vi "Get Excess TempProtection Setpoint.vi"(8 "error in (no error)":errorcluster, 11 "VISA resource name":refnum<visa-resource-name>) -> (0 "error out":errorcluster, 1 "ExcessTempProtection(out)":dbl, 3 "VISA resource name out":refnum<visa-resource-name>)   [LabVIEW 2018, in "JULABO DeviceDriver.lvlib"]
doc: "This VI returns the actual setting for the excess temperature protection. Please refer to operating manual for this safety setting."
uses:
  JULABO DeviceDriver.lvlib
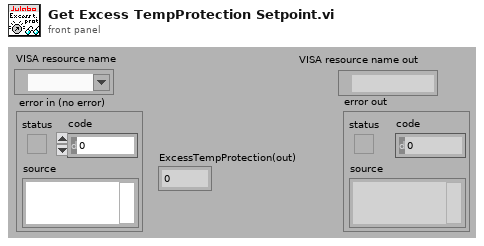
[diagram p1: front panel]
types:
  T1 = typedef "JULABO DeviceDriver.lvlib/InstrumentType.ctl" = enum8{"Default", "FC-Series", "HT30/HT60", "LC4"}
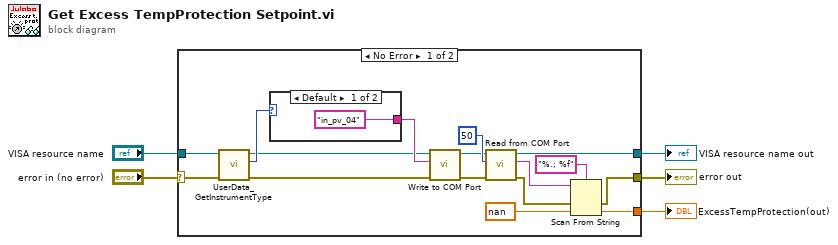
[diagram p0: block diagram]
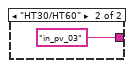
[diagram p2: hidden frame]
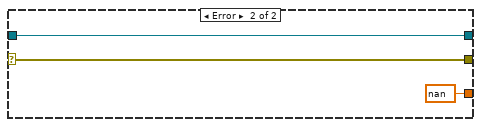
[diagram p3: hidden frame]
diagram:
  n1 = case shown="No Error" "error in (no error)" {
    selector: "error in (no error)" -> [w6 w25]
    tunnel: "VISA resource name" -> [w7 w26]
    tunnel: [w18 w25] -> w4
    tunnel: [w17 w26] -> w3
    tunnel: [w15 nan] -> w1
    frame No Error {
      n2 = call "UserData_GetInstrumentType.vi"("Fehler (Eingang)"=w6, "VISA resource name in"=w7) -> ("Fehler (Ausgang)"=w11:errorcluster, "InstrumentType"=w12:T1, "VISA resource name out"=w10:refnum<visa-resource-name>)  [unwired: 3 in]
      n3 = case shown="Default" w12 {
        tunnel: ["in_pv_04" "in_pv_03"] -> w13
        frame Default {
        }
        frame "HT30/HT60" {
        }
      }
      n4 = call "Write to COM Port.vi"("error in"=w11, "Command (input)"=w13, "VISA resource name in"=w10) -> ("error out"=w8:errorcluster, "VISA resource name out"=w9:refnum<visa-resource-name>)  [unwired: 7 in]
      n5 = call "Read from COM Port.vi"("error in"=w8, "Byte to Read (-1:All)"=50 ("Anzahl der Byte"), "VISA resource name in"=w9) -> ("error out"=w20:errorcluster, "String (output)"=w19:string, "VISA resource name out"=w17:refnum<visa-resource-name>)  [unwired: 5 in, 1 out]
      n6 = Scan From String(format string="%.; %f" ("Format-String"), input string=w19, error in=w20, default 1=nan ("Standardwert1")) -> (error out=w18:errorcluster, output 1=w15:dbl)  [unwired: 1 in, 2 out]
    }
    frame Error {
    }
  }
  "error out" <- w4
  "VISA resource name out" <- w3
  "ExcessTempProtection(out)" <- w1
